vi "ex_RemoveSpecialFromChunk.vi"(8 "error in (no error)":errorcluster, 11 "chunk in":string) -> (0 "error out":errorcluster, 1 "no special?":bool, 2 "special blocks":string[](array[string]), 3 "chunk remainder":string, 4 "partial special?":bool)   [LabVIEW 2017]
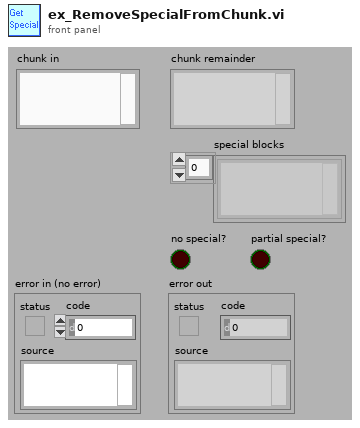
[diagram p1: front panel]
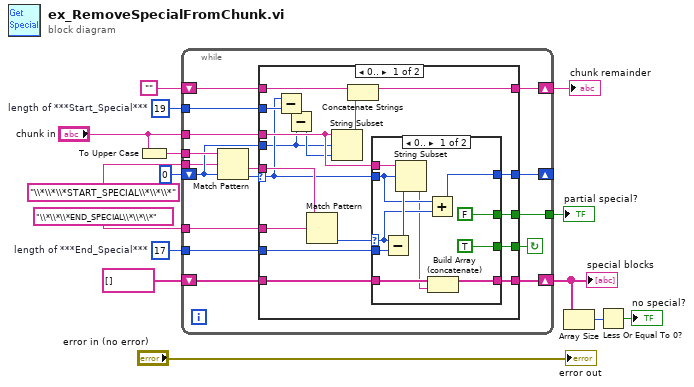
[diagram p0: block diagram]
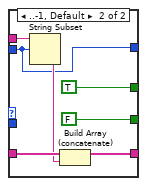
[diagram p2: hidden frame]
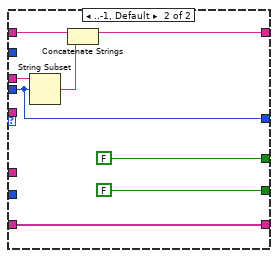
[diagram p3: hidden frame]
diagram:
  w11 = 19  # length of ***Start_Special***
  w1 = 17  # length of ***End_Special***
  n1 = To Upper Case(1:"chunk in") -> (0:w15:string)
  n2 = while {
    tunnel: w15 -> [w31]
    shift-right: [w17] -> w6
    shift-left: string[] [] ("special blocks") -> [w18]
    tunnel: "chunk in" -> [w28]
    shift-right: [w20] -> w9
    shift-left: "" -> [w27]
    shift-right: [w21] -> _
    shift-left: 0 ("offset (0)") -> [w26]
    tunnel: w11 -> [w25]
    tunnel: "\\*\\*\\*START_SPECIAL\\*\\*\\*" -> [w24]
    tunnel: w1 -> [w23]
    tunnel: "\\*\\*\\*END_SPECIAL\\*\\*\\*" -> [w22]
    tunnel: [w16] -> w3
    stop <- w19 continue-if-true
    n3 = Match Pattern(string=w31, regular expression=w24, offset (0)=w26) -> (after substring=w29:string, offset past match=w30:i32)  [unwired: 2 out]
    n4 = case shown="0.." w30 {
      selector: w30 -> [w33 _]
      tunnel: w29 -> [w45 _]
      tunnel: w28 -> [w48 w72]
      tunnel: w27 -> [w49 w75]
      tunnel: w26 -> [w32 w71]
      tunnel: w25 -> [w44 _]
      tunnel: w23 -> [w35 _]
      tunnel: w22 -> [w46 _]
      tunnel: [w36 w71] -> w21
      tunnel: [w41 w74] -> w20
      tunnel: [w40 FALSE] -> w19
      tunnel: w18 -> [w39 w69]
      tunnel: [w38 w69] -> w17
      tunnel: [w37 FALSE] -> w16
      frame 0.. {
        n5 = Subtract(x=w33, y=w44) -> (x-y=w43:i32)
        n6 = Subtract(x=w43, y=w32) -> (x-y=w34:i32)
        n7 = Match Pattern(string=w45, regular expression=w46) -> (offset past match=w42:i32)  [unwired: 4 out]
        n8 = String Subset(string=w48, offset (0)=w32, length (rest)=w34) -> (substring=w47:string)
        n9 = Concatenate Strings(w49, w47) -> (w41:string)
        n10 = case shown="0.." w42 {
          selector: w42 -> [w57 _]
          tunnel: w48 -> [w60 w66]
          tunnel: [TRUE FALSE] -> w40
          tunnel: w33 -> [w56 w61]
          tunnel: w39 -> [w54 w65]
          tunnel: [w52 w64] -> w38
          tunnel: [FALSE TRUE] -> w37
          tunnel: [w55 w61] -> w36
          tunnel: w35 -> [w59 _]
          frame 0.. {
            n11 = Subtract(x=w57, y=w59) -> (x-y=w58:i32)
            n12 = String Subset(string=w60, offset (0)=w56, length (rest)=w58) -> (substring=w53:string)
            n13 = Add(x=w56, y=w57) -> (x+y=w55:i32)
            n14 = Build Array (concatenate)(w54, w53) -> (w52:string[])
          }
          frame ..-1, Default {
            n15 = String Subset(string=w66, offset (0)=w61) -> (substring=w63:string)  [unwired: 1 out]
            n16 = Build Array (concatenate)(w65, w63) -> (w64:string[])
          }
        }
      }
      frame ..-1, Default {
        n17 = String Subset(string=w72, offset (0)=w71) -> (substring=w73:string)  [unwired: 1 out]
        n18 = Concatenate Strings(w75, w73) -> (w74:string)
      }
    }
  }
  "chunk remainder" <- w9
  "special blocks" <- w6
  "partial special?" <- w3
  n19 = Array Size(array=w6) -> (size(s)=w5:i32)
  n20 = Less Or Equal To 0?(x=w5) -> (x <= 0?=→"no special?":bool)
  "error out" <- "error in (no error)"
